vi "searchNode.vi"(8 "error in (no error)":errorcluster, 9 "searchXPath":string, 11 "NativeXML in":refnum<class "NativeXML.lvclass">) -> (0 "error out":errorcluster, 2 "nodeArray":refnum<class "NativeXML.lvclass">[](array[class]), 3 "NativeXML out":refnum<class "NativeXML.lvclass">)   [LabVIEW 2009, in "Tools.lvlib" / "xml.lvlib" / "NativeXML.lvclass"]
uses:
  NativeXML.lvclass
  NativeXML.lvclass/NativeXML.ctl
  <vilib>/xml/NI_XML.lvlib
panel:
  in  "searchElementIn":string
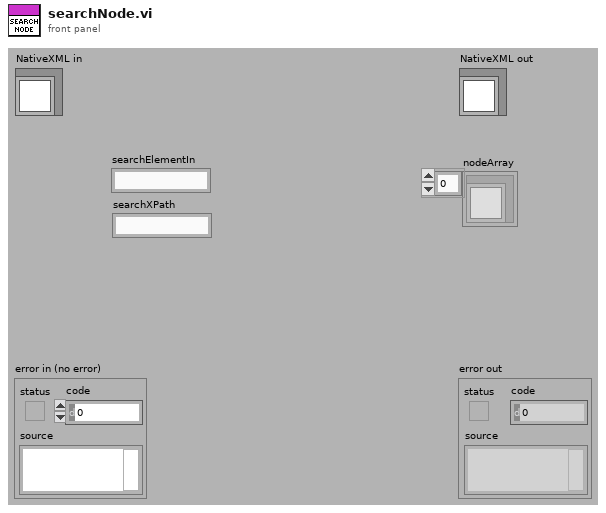
[diagram p1: front panel]
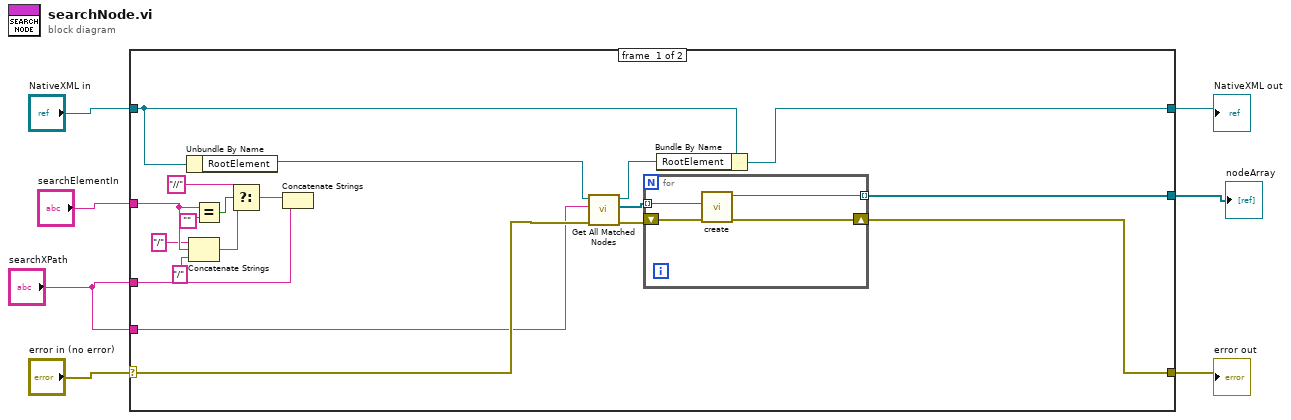
[diagram p0: block diagram]
diagram:
  n1 = case shown="No Error" "error in (no error)" {
    selector: "error in (no error)" -> [w10 w32]
    tunnel: [w24 w32] -> w6
    tunnel: [w25 w31] -> w4
    tunnel: "NativeXML in" -> [w26 w31]
    tunnel: "searchElementIn" -> [w19 _]
    tunnel: "searchXPath" -> [w16 _]
    tunnel: [w9 _] -> w2
    tunnel: "searchXPath" -> [w8 _]
    frame #0 {
      n2 = Unbundle By Name(w26) -> ("RootElement"=w11:refnum<k20>)
      n3 = Concatenate Strings("/", w19, "/") -> (w20:string)
      n4 = Equal?(x=w19, y="") -> (x = y?=w23:bool)
      n5 = Select(t="//", s=w23, f=w20) -> (s? t:f=w17:string)
      n6 = Concatenate Strings(w17, w16) -> ()  [unwired: 1 out]
      n7 = call <vilib>:"Get All Matched Nodes.vi"("error in (no error)"=w10, "XPath expression"=w8, "node in"=w11) -> ("error out"=w13:errorcluster, "node result array"=w14:refnum<k20>[], "node out"=w12:refnum<k20>)  [unwired: 6 in]
      n8 = for {
        tunnel: w14 -> [w29] mode=indexing
        tunnel: [w28] -> w9 mode=indexing
        shift-right: [w27] -> w24
        shift-left: w13 -> [w30]
        n9 = call "create.vi"("error in (no error)"=w30, "RootElement"=w29) -> ("error out"=w27:errorcluster, "NativeXML out"=w28:refnum<class "NativeXML.lvclass">)  [unwired: 8 in]
      }
      n10 = Bundle By Name(cluster=w26, "RootElement"=w12) -> (w25:refnum<class "NativeXML.lvclass">)
    }
    frame #1 {
    }
  }
  "error out" <- w6
  "NativeXML out" <- w4
  "nodeArray" <- w2
